vi "InitControls.vi"(11 "Config":path) -> ()   [LabVIEW 2012]
uses:
  <vilib>/Utility/config.llb/Read Key (String).vi
  <vilib>/Utility/config.llb/Read Key (U32).vi
  <vilib>/Utility/config.llb/Read Key (Double).vi
  <vilib>/Utility/config.llb/NI_LVConfig.lvlib
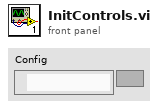
[diagram p1: front panel]
types:
  T1 = typedef "NI_LVConfig.lvlib/Config Data RefNum.ctl" = refnum<k1>
  T2 = cluster{"JoystickRefnum":string, "Axis":u8, "Deadband":dbl}
  T3 = typedef "WPI_JoystickDevRef.ctl" = cluster{"Device":T4}
  T4 = typedef "WPI_JoystickDeviceEnum.ctl" = enum16{"USB 1", "USB 2", "USB 3", "USB 4", "Kinect 1", "Kinect 2"}
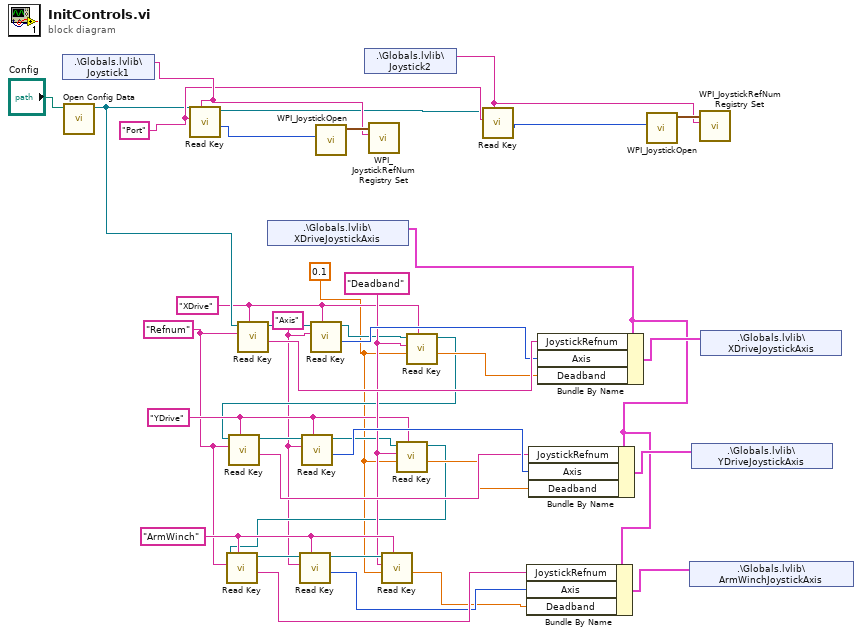
[diagram p0: block diagram]
diagram:
  w3 = 0.1
  w15 = "Deadband"
  w16 = "ArmWinch"
  w10 = "YDrive"
  w5 = "Axis"
  w4 = "Refnum"
  w11 = "XDrive"
  w35 = "Port"
  n1 = shared-variable ".\\Globals.lvlib\\Joystick1"() -> (w36:string)  [unwired: 1 in, 1 out]
  n2 = call <vilib>:"Open Config Data.vi"("configuration file path"="Config") -> ("refnum"=w31:T1)  [unwired: 8 in, 2 out]
  n3 = call-poly <vilib>:"Read Key.vi"("section"=w36, "key"=w35, "refnum"=w31) -> ("value"=w2:u32, "refnum out"=w34:T1)  [unwired: 5 in, 2 out]
  n4 = call-poly <vilib>:"Read Key.vi"("section"=w11, "key"=w4, "refnum"=w31) -> ("value"=w28:string, "refnum out"=w30:T1)  [unwired: 5 in, 2 out]
  n5 = shared-variable ".\\Globals.lvlib\\XDriveJoystickAxis"() -> (w18:T2)  [unwired: 1 in, 1 out]
  n6 = call-poly <vilib>:"Read Key.vi"("section"=w11, "key"=w5, "refnum"=w30) -> ("value"=w27:u32, "refnum out"=w6:T1)  [unwired: 5 in, 2 out]
  n7 = call <vilib>:"WPI_JoystickOpen.vi"("JoystickDevice"=w2) -> ("JoystickDevRef"=w37:T3)  [unwired: 10 in]
  n8 = shared-variable ".\\Globals.lvlib\\Joystick2"() -> (w32:string)  [unwired: 1 in, 1 out]
  n9 = call <vilib>:"WPI_JoystickRefNum Registry Set.vi"("refnum name"=w36, "JoystickDevRef"=w37) -> ()  [unwired: 8 in, 2 out]
  n10 = call-poly <vilib>:"Read Key.vi"("section"=w11, "default value"=w3, "key"=w15, "refnum"=w6) -> ("value"=w12:dbl, "refnum out"=w7:T1)  [unwired: 4 in, 2 out]
  n11 = call-poly <vilib>:"Read Key.vi"("section"=w10, "key"=w4, "refnum"=w7) -> ("value"=w25:string, "refnum out"=w23:T1)  [unwired: 5 in, 2 out]
  n12 = call-poly <vilib>:"Read Key.vi"("section"=w10, "key"=w5, "refnum"=w23) -> ("value"=w26:u32, "refnum out"=w9:T1)  [unwired: 5 in, 2 out]
  n13 = call-poly <vilib>:"Read Key.vi"("section"=w10, "default value"=w3, "key"=w15, "refnum"=w9) -> ("value"=w13:dbl, "refnum out"=w8:T1)  [unwired: 4 in, 2 out]
  n14 = call-poly <vilib>:"Read Key.vi"("section"=w16, "key"=w4, "refnum"=w8) -> ("value"=w20:string, "refnum out"=w22:T1)  [unwired: 5 in, 2 out]
  n15 = call-poly <vilib>:"Read Key.vi"("section"=w16, "key"=w5, "refnum"=w22) -> ("value"=w19:u32, "refnum out"=w17:T1)  [unwired: 5 in, 2 out]
  n16 = call-poly <vilib>:"Read Key.vi"("section"=w16, "default value"=w3, "key"=w15, "refnum"=w17) -> ("value"=w14:dbl)  [unwired: 4 in, 3 out]
  n17 = call-poly <vilib>:"Read Key.vi"("section"=w32, "key"=w35, "refnum"=w34) -> ("value"=w1:u32)  [unwired: 5 in, 3 out]
  n18 = Bundle By Name(cluster=w18, "JoystickRefnum"=w20, "Axis"=w19, "Deadband"=w14) -> (w21:T2)
  n19 = Bundle By Name(cluster=w18, "JoystickRefnum"=w25, "Axis"=w26, "Deadband"=w13) -> (w24:T2)
  n20 = Bundle By Name(cluster=w18, "JoystickRefnum"=w28, "Axis"=w27, "Deadband"=w12) -> (w29:T2)
  n21 = call <vilib>:"WPI_JoystickOpen.vi"("JoystickDevice"=w1) -> ("JoystickDevRef"=w33:T3)  [unwired: 10 in]
  n22 = shared-variable ".\\Globals.lvlib\\ArmWinchJoystickAxis"(w21) -> ()  [unwired: 1 in, 1 out]
  n23 = shared-variable ".\\Globals.lvlib\\YDriveJoystickAxis"(w24) -> ()  [unwired: 1 in, 1 out]
  n24 = call <vilib>:"WPI_JoystickRefNum Registry Set.vi"("refnum name"=w32, "JoystickDevRef"=w33) -> ()  [unwired: 8 in, 2 out]
  n25 = shared-variable ".\\Globals.lvlib\\XDriveJoystickAxis"(w29) -> ()  [unwired: 1 in, 1 out]
